vi "Load Project.vi"(8 "error in (no error)":errorcluster, 10 "Project or Class Path":path, 11 "Project Loader In":refnum<class "Project Loader.lvclass">) -> (0 "error out":errorcluster, 3 "Project Loader Out":refnum<class "Project Loader.lvclass">)   [LabVIEW 2020, in "Project Loader.lvclass"]
uses:
  Project Loader.lvclass
  Project Loader.lvclass/Project Loader.ctl
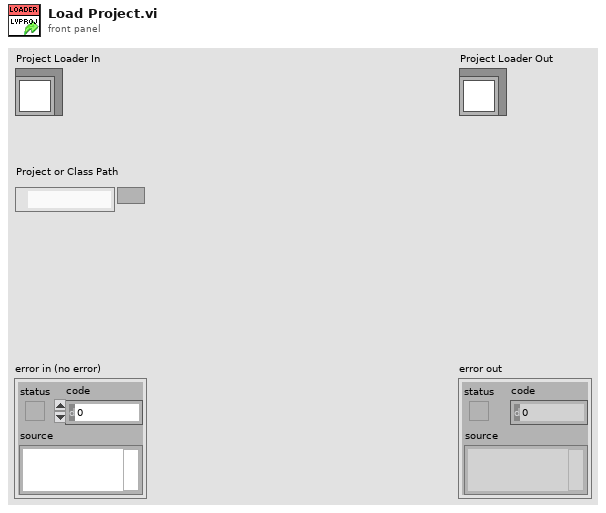
[diagram p1: front panel]
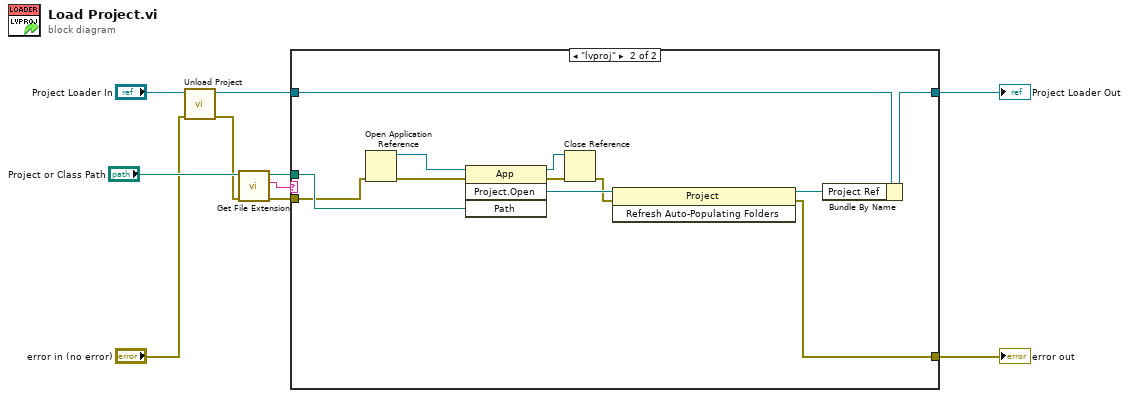
[diagram p0: block diagram]
diagram:
  n1 = call "Unload Project.vi"("error in (no error)"="error in (no error)", "Project Loader In"="Project Loader In") -> ("error out"=w2:errorcluster, "Project Loader Out"=w3:refnum<class "Project Loader.lvclass">)  [unwired: 8 in]
  n2 = call <vilib>:"Get File Extension.vi"("error in (no error)"=w2, "file"="Project or Class Path") -> ("error out"=w7:errorcluster, "lowercase file extension"=w5:string, "dup file"=w9:path)  [unwired: 5 in, 2 out]
  n3 = case shown="\"lvproj\"" w5 {
    tunnel: w3 -> [w12 w24]
    tunnel: w9 -> [_ w19]
    tunnel: [w12 w18] -> w8
    tunnel: w7 -> [w11 w14]
    tunnel: [w11 w13] -> w6
    frame Default {
    }
    frame "lvproj" {
      n4 = Open Application Reference(8:w14) -> (0:w21:errorcluster, 3:w20:refnum<vi>)  [unwired: 3 in]
      n5 = invoke class="App" method="Project.Open"(reference=w20, error in=w21, "Path"=w19) -> (reference out=w23:refnum<vi>, error out=w22:errorcluster, "Project:Open"=w17:refnum<vi>)  [unwired: 1 in, 1 out]
      n6 = Close Reference(reference=w23, error in (no error)=w22) -> (error out=w15:errorcluster)
      n7 = invoke class="Project" method="Refresh Auto-Populating Folders"(reference=w17, error in=w15) -> (reference out=w16:refnum<vi>, error out=w13:errorcluster)  [unwired: 1 in, 1 out]
      n8 = Bundle By Name(cluster=w24, "Project Ref"=w16) -> (w18:refnum<class "Project Loader.lvclass">)
    }
  }
  "error out" <- w6
  "Project Loader Out" <- w8
